vi "niRFUtil RFHS Benchmark Mgr GetTreeBranch.vi"(0 "Tree":T1[](array[typedef]), 5 "Owner":u32) -> (4 "Branch":T1[](array[typedef]))   [LabVIEW 2015, in "niRFUtil.lvlib"]
uses:
  niRFUtil.lvlib
  niRFUtil RFHS Benchmark TaskMgrInfo.ctl
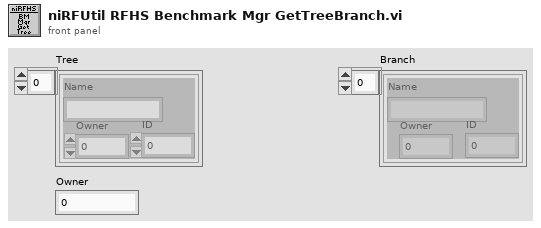
[diagram p1: front panel]
types:
  T1 = typedef "niRFUtil.lvlib/niRFUtil RFHS Benchmark TaskMgrInfo.ctl" = cluster{"Name":string, "Owner":i32, "ID":i32}
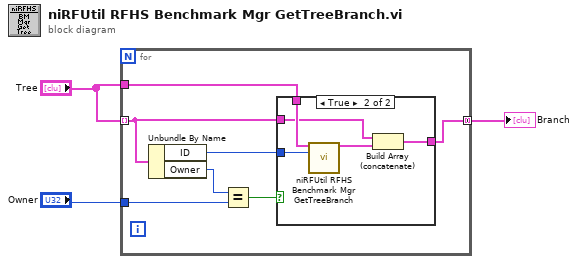
[diagram p0: block diagram]
diagram:
  n1 = for {
    tunnel: "Tree" -> [w4] mode=indexing
    tunnel: "Owner" -> [w9]
    tunnel: "Tree" -> [w8]
    tunnel: [w7] -> w3 mode=concatenating
    n2 = Unbundle By Name(w4) -> ("ID"=w5:i32, "Owner"=w10:i32)
    n3 = Equal?(x=w10, y=w9) -> (x = y?=w6:bool)
    n4 = case shown="True" w6 {
      tunnel: w8 -> [_ w15]
      tunnel: [_ w12] -> w7
      tunnel: w5 -> [_ w13]
      tunnel: w4 -> [_ w11]
      frame False {
      }
      frame True {
        n5 = call "niRFUtil RFHS Benchmark Mgr GetTreeBranch.vi"("Tree"=w15, "Owner"=w13) -> ("Branch"=w14:T1[])  [unwired: 13 in]
        n6 = Build Array (concatenate)(w11, w14) -> (w12:T1[])
      }
    }
  }
  "Branch" <- w3
